vi "dvp Vi Is Online.vi"(10 "pIsOnline":i32, 11 "handle":u32) -> (2 "pIsOnline out":i32, 3 "function return":u32(ring))   [LabVIEW 2018, in "LabViewDVPCamera.lvlib"]
doc: "LabviewDvp2Api dvpStatus dvpViIsOnline(dvpHandle handle, BOOL *pIsOnline);"
uses:
  LabViewDVPCamera.lvlib
  LabViewDVPCamera/LabViewDVPCamera.dll
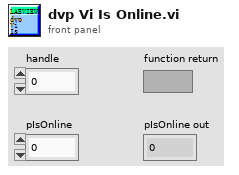
[diagram p1: front panel]
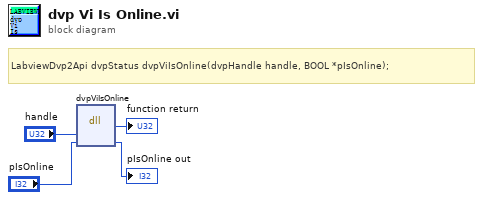
[diagram p0: block diagram]
diagram:
  # "LabviewDvp2Api dvpStatus dvpViIsOnline(dvpHandle handle, BOOL *pIsOnline);"
  n1 = dll-call lib="C:/Program Files (x86)/DVP2 Labview cn 64/Sample/LabViewDVPCamera/LabViewDVPCamera.*" fn="dvpViIsOnline"("handle"="handle", "pIsOnline"="pIsOnline") -> (→"function return":u32, "pIsOnline"=→"pIsOnline out":i32)  [unwired: 4 in, 2 out]
